vi "Write Text File.vi"(8 "error in":errorcluster, 9 "Number of Samples":i32, 10 "Data In":dbl[][](array[numeric]) format="%0.2f", 11 "File Path":path) -> (0 "error out":errorcluster)   [LabVIEW 2021]
panel:
  out "Data In 2":dbl[][](array[numeric])
  out "spreadsheet string":string
  out "Format string 2":string
  out "Header string":string
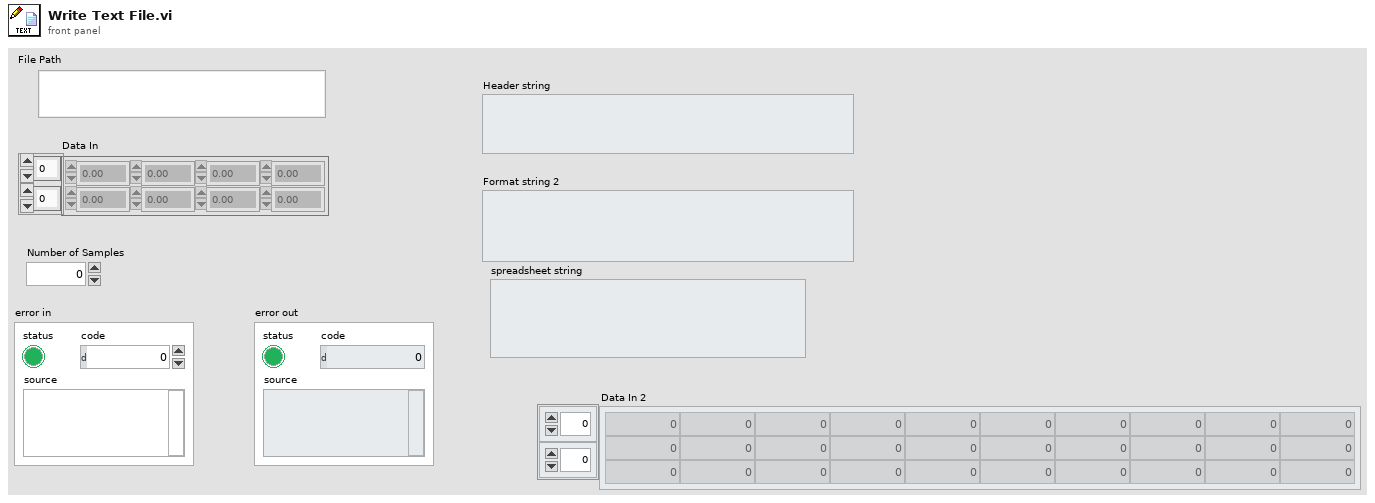
[diagram p1: front panel]
types:
  T1 = enum16{"open", "replace", "create", "open or create", "replace or create", "replace or create with confirmation"}
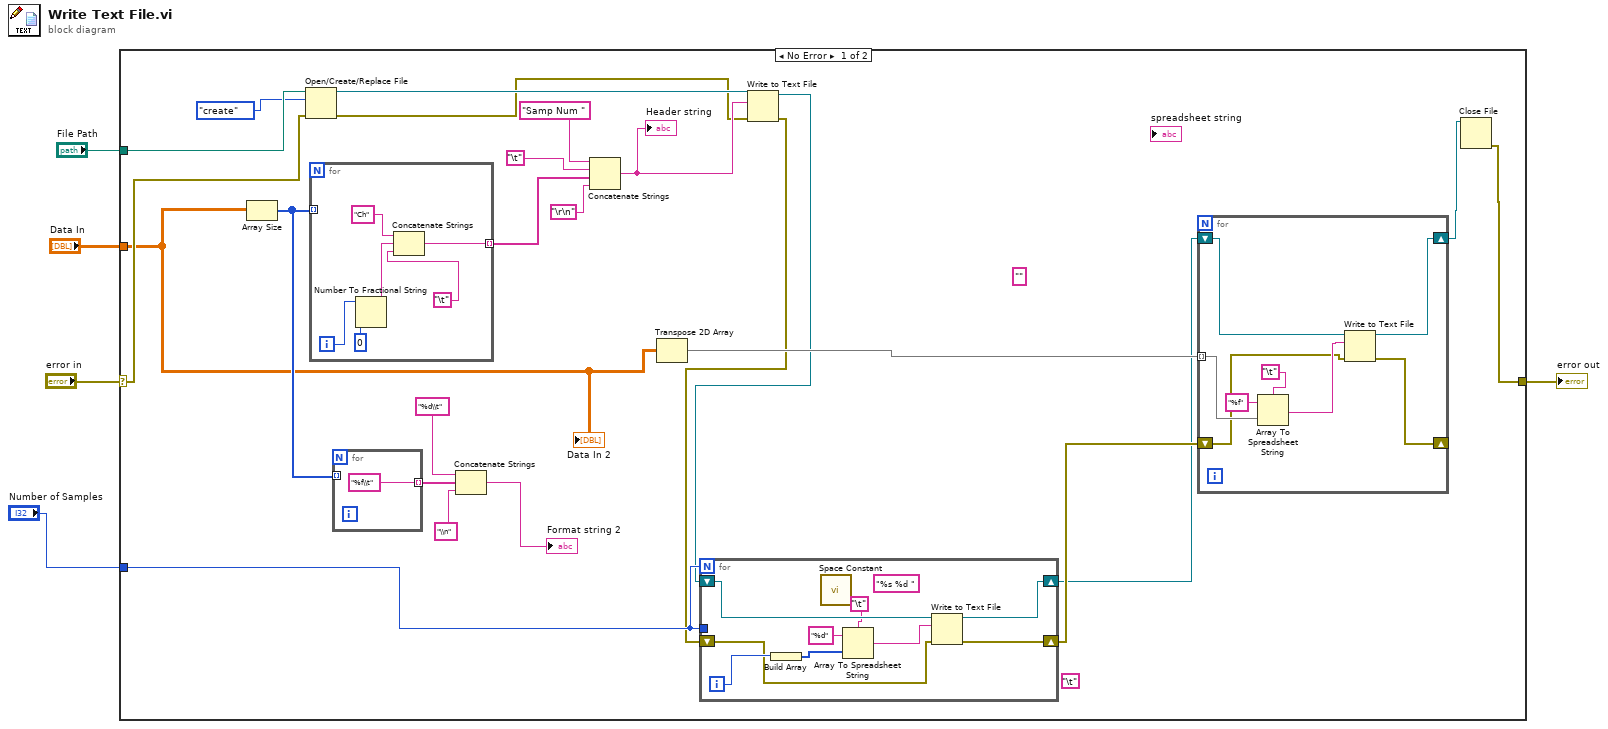
[diagram p0: block diagram]
diagram:
  n1 = case shown="No Error" "error in" {
    selector: "error in" -> [w16 w54]
    tunnel: "Data In" -> [w11 _]
    tunnel: "File Path" -> [w23 _]
    tunnel: [w14 w54] -> w2
    tunnel: "Number of Samples" -> [w10 _]
    frame No Error {
      (unwired) "\t"
      (unwired) "" ("spreadsheet string")
      n2 = Array Size(array=w11) -> (size(s)=w24:i32[])
      n3 = Open/Create/Replace File(file path (use dialog)=w23, error in=w16, operation (0:open)=T1."create") -> (refnum out=w21:refnum<file>, error out=w15:errorcluster)  [unwired: 3 in, 1 out]
      n4 = for {
        tunnel: w24 -> [_] mode=indexing
        tunnel: [w50] -> w18 mode=indexing
        i -> [w52]
        n5 = Number To Fractional String(number=w52, precision (6)=i16 0) -> (F-format string=w51:string)  [unwired: 2 in]
        n6 = Concatenate Strings("Ch" ("string"), w51, "\t") -> (w50:string)
      }
      n7 = for {
        tunnel: w24 -> [_] mode=indexing
        tunnel: ["%f\\t" ("string")] -> w26 mode=indexing
      }
      n8 = Concatenate Strings("%d\\t", w26, "\\n" ("string")) -> (→"Format string 2":string)
      n9 = Concatenate Strings("Samp Num ", "\t", w18, "\r\n") -> (w20:string)
      "Header string" <- w20
      n10 = Transpose 2D Array(2D array=w11) -> (transposed array=w13:dbl[][])
      n11 = Write to Text File(file (use dialog)=w21, text=w20, error in=w15) -> (refnum out=w9:refnum<file>, error out=w8:errorcluster)  [unwired: 1 in, 1 out]
      n12 = for {
        N: w10 -> [_]
        tunnel: w10 -> [_]
        shift-right: [w37] -> w6
        shift-left: w9 -> [w38]
        shift-right: [w36] -> w7
        shift-left: w8 -> [w30]
        i -> [w35]
        (unwired) "%s %d " ("format string")
        n13 = Build Array(w35) -> (w34:i32[])
        n14 = call <vilib>:"Space Constant.vi"() -> ()  [unwired: 1 out]
        n15 = Array To Spreadsheet String(delimiter (Tab)="\t", array=w34, 3:"%d" ("format string")) -> (spreadsheet string=w31:string)
        n16 = Write to Text File(file (use dialog)=w38, text=w31, error in=w30) -> (refnum out=w37:refnum<file>, error out=w36:errorcluster)  [unwired: 1 in, 1 out]
      }
      n17 = for {
        tunnel: w13 -> [w45] mode=indexing
        shift-right: [w42] -> w12
        shift-left: w6 -> [w43]
        shift-right: [w40] -> _
        shift-left: w7 -> [w41]
        n18 = Array To Spreadsheet String(delimiter (Tab)="\t", array=w45, 3:"%f" ("format string")) -> (spreadsheet string=w44:string)
        n19 = Write to Text File(file (use dialog)=w43, text=w44, error in=w41) -> (refnum out=w42:refnum<file>, error out=w40:errorcluster)  [unwired: 1 in, 1 out]
      }
      n20 = Close File(refnum=w12) -> (error out=w14:errorcluster)  [unwired: 1 in, 1 out]
      "Data In 2" <- w11
    }
    frame Error {
    }
  }
  "error out" <- w2
